vi "Write Channel Status.vi"(8 "error in (no error)":errorcluster, 10 "Channel Status":map{string, T1}(c390), 11 "CIFCorePlugin in":refnum<class "CIFCorePlugin.lvclass">) -> (0 "error out":errorcluster, 3 "CIFCorePlugin out":refnum<class "CIFCorePlugin.lvclass">)   [LabVIEW 2021, in "CIFCorePlugin.lvclass"]
uses:
  CIFCorePlugin.lvclass
  CIFUtilities/CIFChannelMng/typedef/Channel List for OOB.ctl
  CIFUtilities/CIFChannels/Typedef/Direction.ctl
  CIFCorePlugin.lvclass/CIFCorePlugin.ctl
  CIFUtilities/CIFChannelMng/CIFChannelMng.lvclass/CIFChannelMng.ctl
  CIFUtilities/CIFChannelMng/CIFChannelMng.lvclass
  CIFUtilities/CIFChannels/CIFChannels.lvclass
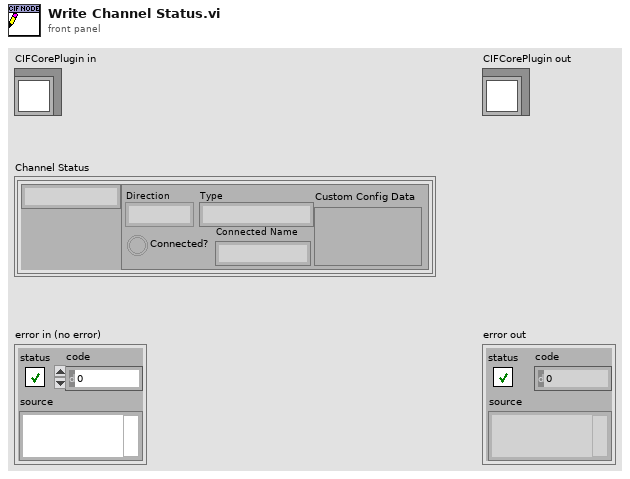
[diagram p1: front panel]
types:
  T1 = typedef "CIFChannelMng.lvclass/Channel List for OOB.ctl" = cluster{"Direction":T2, "Type":string, "Custom Config Data":variant, "Connected?":bool, "Connected Name":string}
  T2 = typedef "CIFChannels.lvclass/Direction.ctl" = enum16{"Publisher", "Subscriber"}
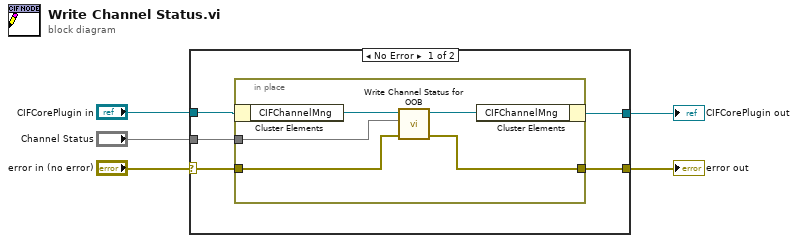
[diagram p0: block diagram]
diagram:
  n1 = case shown="No Error" "error in (no error)" {
    selector: "error in (no error)" -> [w7 w16]
    tunnel: [w6 w16] -> w4
    tunnel: [w8 w17] -> w2
    tunnel: "CIFCorePlugin in" -> [w9 w17]
    tunnel: "Channel Status" -> [w10 _]
    frame No Error {
      n2 = in-place {
        in-place-border: w10 -> [w15]
        in-place-border: w7 -> [w12]
        in-place-border: [w11] -> w6
        n3 = in-place-cluster #1(w9) -> ("CIFChannelMng"=w14:refnum<class "CIFChannelMng.lvclass">)
        n4 = call "Write Channel Status for OOB.vi"("error in (no error)"=w12, "Channel Status for OOB"=w15, "CIFChannelMng in"=w14) -> ("error out"=w11:errorcluster, "CIFChannelMng out"=w13:refnum<class "CIFChannelMng.lvclass">)  [unwired: 7 in]
        n5 = in-place-cluster #1("CIFChannelMng"=w13) -> (w8:refnum<class "CIFCorePlugin.lvclass">)
      }
    }
    frame Error {
    }
  }
  "error out" <- w4
  "CIFCorePlugin out" <- w2
